vi "rep-worker.vi"() -> ()   [LabVIEW 2014]
uses:
  <vilib>/addons/zeromq/socket_type.ctl
  <vilib>/addons/zeromq/zmq_context.lvclass
  <vilib>/addons/zeromq/zeromq.lvlib
  <vilib>/addons/zeromq/zmq_socket.lvclass
panel:
  out "concatenated string":string
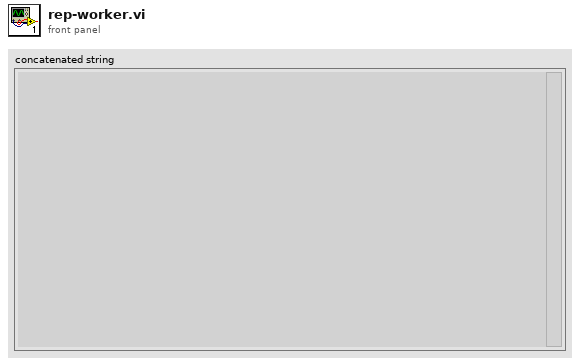
[diagram p1: front panel]
types:
  T1 = typedef "zeromq.lvlib/socket_type.ctl" = enum8{"ZMQ_PAIR", "ZMQ_PUB", "ZMQ_SUB", "ZMQ_REQ", "ZMQ_REP", "ZMQ_DEALER", "ZMQ_ROUTER", "ZMQ_PULL", "ZMQ_PUSH", "ZMQ_XPUB", "ZMQ_XSUB"}
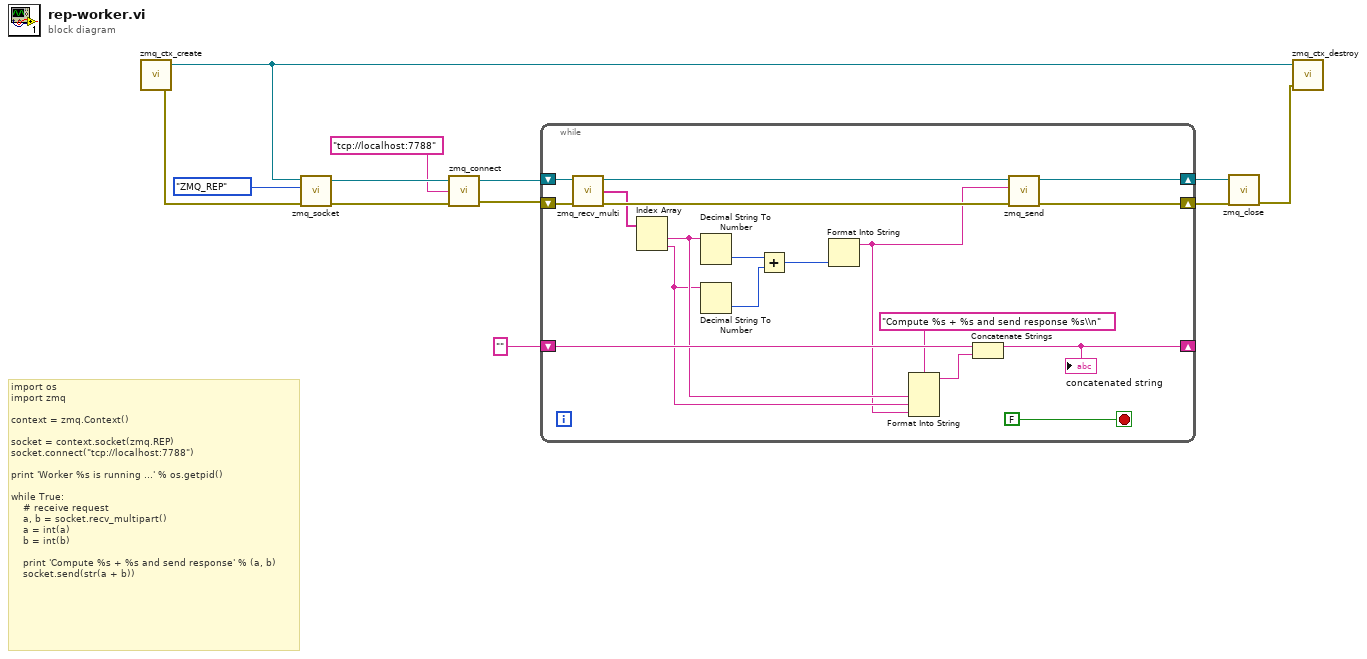
[diagram p0: block diagram]
diagram:
  # "import os\nimport zmq\n\ncontext = zmq.Context()\n\nsocket = context.socket(zmq.REP)\nsocket.connect(\"tcp://localhost:7788\")\n\nprint 'Worker %s is running ...' % os.getpid()\n\nwhile True:\n    # receive request\n    a, b = socket.recv_multipart()\n    a = int(a)\n    b = int(b)\n\n    print 'Compute %s + %s and send response' % (a, b)\n    socket.send(str(a + b))"
  n1 = call <vilib>:"zmq_ctx_create.vi"() -> ("error out"=w11:errorcluster, "context out"=w10:refnum<class "zmq_context.lvclass">)  [unwired: 4 in]
  n2 = call <vilib>:"zmq_socket.vi"("error in"=w11, "socket type"=socket_type."ZMQ_REP", "context in"=w10) -> ("error out"=w8:errorcluster, "socket out"=w9:refnum<class "zmq_socket.lvclass">)  [unwired: 2 in, 1 out]
  n3 = call <vilib>:"zmq_connect.vi"("error in"=w8, "endpoint"="tcp://localhost:7788", "socket in"=w9) -> ("error out"=w5:errorcluster, "socket out"=w6:refnum<class "zmq_socket.lvclass">)  [unwired: 1 in]
  n4 = while {
    shift-right: [w26] -> w4
    shift-left: w6 -> [w30]
    shift-right: [w25] -> w3
    shift-left: w5 -> [w29]
    shift-right: [w14] -> _
    shift-left: "" -> [w19]
    stop <- FALSE stop-if-true
    n5 = call <vilib>:"zmq_recv_multi.vi"("error in"=w29, "socket in"=w30) -> ("error out"=w27:errorcluster, "parts"=w24:string[], "socket out"=w28:refnum<class "zmq_socket.lvclass">)  [unwired: 1 in]
    n6 = Index Array(array=w24) -> (element #1=w18:string, element #2=w17:string)  [unwired: 2 in]
    n7 = Decimal String To Number(string=w18) -> (number=w23:i32)  [unwired: 2 in, 1 out]
    n8 = Decimal String To Number(string=w17) -> (number=w22:i32)  [unwired: 2 in, 1 out]
    n9 = Add(x=w23, y=w22) -> (x+y=w20:i32)
    n10 = Format Into String(w20) -> (resulting string=w16:string)  [unwired: 3 in, 1 out]
    n11 = Format Into String(format string="Compute %s + %s and send response %s\\n", w18, w17, w16) -> (resulting string=w13:string)  [unwired: 2 in, 1 out]
    n12 = Concatenate Strings(w19, w13) -> (w14:string)
    "concatenated string" <- w14
    n13 = call <vilib>:"zmq_send.vi"("error in"=w27, "data"=w16, "socket in"=w28) -> ("error out"=w25:errorcluster, "socket out"=w26:refnum<class "zmq_socket.lvclass">)  [unwired: 4 in]
  }
  n14 = call <vilib>:"zmq_close.vi"("error in"=w3, "socket"=w4) -> ("error out"=w2:errorcluster)  [unwired: 3 in]
  n15 = call <vilib>:"zmq_ctx_destroy.vi"("error in"=w2, "context in"=w10) -> ()  [unwired: 3 in, 1 out]
